vi "PPS_TRAJECTORY_DASH_WRITE.vi"   [LabVIEW 2019]
uses:
  PPS_TRAJECTORY_GLOBALS.vi
  <vilib>/Rock Robotics/Network Tables/NT Write Number.vi
  <vilib>/Rock Robotics/Network Tables/NT Write Boolean.vi
  <vilib>/Rock Robotics/Network Tables/NT Write Numeric Array.vi
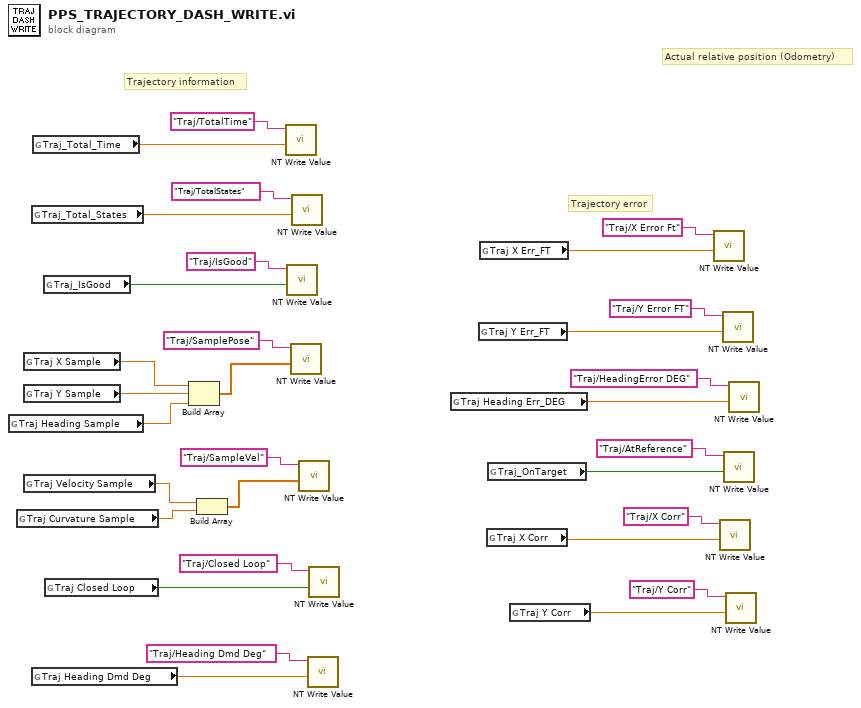
[diagram p0: block diagram]
diagram:
  # "Trajectory information"
  # "Actual relative position (Odometry)"
  # "Trajectory error"
  n1 = global read "PPS_TRAJECTORY_GLOBALS.vi" "Traj Heading Sample"() -> (w11:dbl)
  n2 = global read "PPS_TRAJECTORY_GLOBALS.vi" "Traj Curvature Sample"() -> (w9:dbl)
  n3 = global read "PPS_TRAJECTORY_GLOBALS.vi" "Traj X Sample"() -> (w13:dbl)
  n4 = global read "PPS_TRAJECTORY_GLOBALS.vi" "Traj Y Sample"() -> (w12:dbl)
  n5 = global read "PPS_TRAJECTORY_GLOBALS.vi" "Traj Velocity Sample"() -> (w10:dbl)
  n6 = global read "PPS_TRAJECTORY_GLOBALS.vi" "Traj_Total_States"() -> (w15:dbl)
  n7 = global read "PPS_TRAJECTORY_GLOBALS.vi" "Traj Heading Dmd Deg"() -> (w7:dbl)
  n8 = global read "PPS_TRAJECTORY_GLOBALS.vi" "Traj_Total_Time"() -> (w14:dbl)
  n9 = global read "PPS_TRAJECTORY_GLOBALS.vi" "Traj_IsGood"() -> (w16:bool)
  n10 = global read "PPS_TRAJECTORY_GLOBALS.vi" "Traj Closed Loop"() -> (w8:bool)
  n11 = Build Array(w13, w12, w11) -> (w25:dbl[])
  n12 = Build Array(w10, w9) -> (w27:dbl[])
  n13 = call-poly <vilib>:"NT Write Value.vi"("value"=w14, "name"="Traj/TotalTime" ("Name")) -> ()  [unwired: 9 in, 1 out]
  n14 = call-poly <vilib>:"NT Write Value.vi"("value"=w16, "name"="Traj/IsGood" ("Name")) -> ()  [unwired: 9 in, 1 out]
  n15 = call-poly <vilib>:"NT Write Value.vi"("value"=w25, "name"="Traj/SamplePose" ("Name")) -> ()  [unwired: 9 in, 1 out]
  n16 = call-poly <vilib>:"NT Write Value.vi"("value"=w15, "name"="Traj/TotalStates" ("Name")) -> ()  [unwired: 9 in, 1 out]
  n17 = call-poly <vilib>:"NT Write Value.vi"("value"=w27, "name"="Traj/SampleVel" ("Name")) -> ()  [unwired: 9 in, 1 out]
  n18 = call-poly <vilib>:"NT Write Value.vi"("value"=w7, "name"="Traj/Heading Dmd Deg" ("Name")) -> ()  [unwired: 9 in, 1 out]
  n19 = call-poly <vilib>:"NT Write Value.vi"("value"=w8, "name"="Traj/Closed Loop" ("Name")) -> ()  [unwired: 9 in, 1 out]
  n20 = global read "PPS_TRAJECTORY_GLOBALS.vi" "Traj Heading Err_DEG"() -> (w4:dbl)
  n21 = global read "PPS_TRAJECTORY_GLOBALS.vi" "Traj Y Err_FT"() -> (w6:dbl)
  n22 = global read "PPS_TRAJECTORY_GLOBALS.vi" "Traj X Err_FT"() -> (w5:dbl)
  n23 = global read "PPS_TRAJECTORY_GLOBALS.vi" "Traj X Corr"() -> (w1:dbl)
  n24 = global read "PPS_TRAJECTORY_GLOBALS.vi" "Traj_OnTarget"() -> (w3:bool)
  n25 = global read "PPS_TRAJECTORY_GLOBALS.vi" "Traj Y Corr"() -> (w2:dbl)
  n26 = call-poly <vilib>:"NT Write Value.vi"("value"=w5, "name"="Traj/X Error Ft" ("Name")) -> ()  [unwired: 9 in, 1 out]
  n27 = call-poly <vilib>:"NT Write Value.vi"("value"=w1, "name"="Traj/X Corr" ("Name")) -> ()  [unwired: 9 in, 1 out]
  n28 = call-poly <vilib>:"NT Write Value.vi"("value"=w6, "name"="Traj/Y Error FT" ("Name")) -> ()  [unwired: 9 in, 1 out]
  n29 = call-poly <vilib>:"NT Write Value.vi"("value"=w3, "name"="Traj/AtReference" ("Name")) -> ()  [unwired: 9 in, 1 out]
  n30 = call-poly <vilib>:"NT Write Value.vi"("value"=w2, "name"="Traj/Y Corr" ("Name")) -> ()  [unwired: 9 in, 1 out]
  n31 = call-poly <vilib>:"NT Write Value.vi"("value"=w4, "name"="Traj/HeadingError DEG" ("Name")) -> ()  [unwired: 9 in, 1 out]
